vi "DCIR_run_1pulseGene.vi"(6 "3P4S":bool, 7 "Offset%":sgl, 8 "errin":errorcluster, 9 "AmpCharg":dbl, 11 "VisaAlimIn":refnum<visa-resource-name>) -> (0 "errout":errorcluster, 1 "PV":string, 2 "DATAout":cluster{"Rch":dbl, "A ch":dbl, "max":dbl}, 3 "VisaAlimOut":refnum<visa-resource-name>, 4 "Out":T1, 5 "Cell et DCIR ok":bool)   [LabVIEW 2020]
uses:
  <userlib>/PCAN Basic/Controls/BaudrateEenum.ctl
  <userlib>/PCAN Basic/Controls/Channel.ctl
  Param_Stack.vi
  ctrl glo/VG_progressBar.vi
  <instrlib>/IT6000C/IT6000C.lvlib
  <userlib>/Alex_Peak_lib/PEAK_lib_ALEX.lvlib
  <userlib>/PCAN Basic/PCANBasic.lvlib
panel:
  out "isPASS?":bool
  out "Rcharge":dbl
  out "Rmax":dbl
  out "V gamme":bool
  in  "stop":bool
  out "Booléen":bool
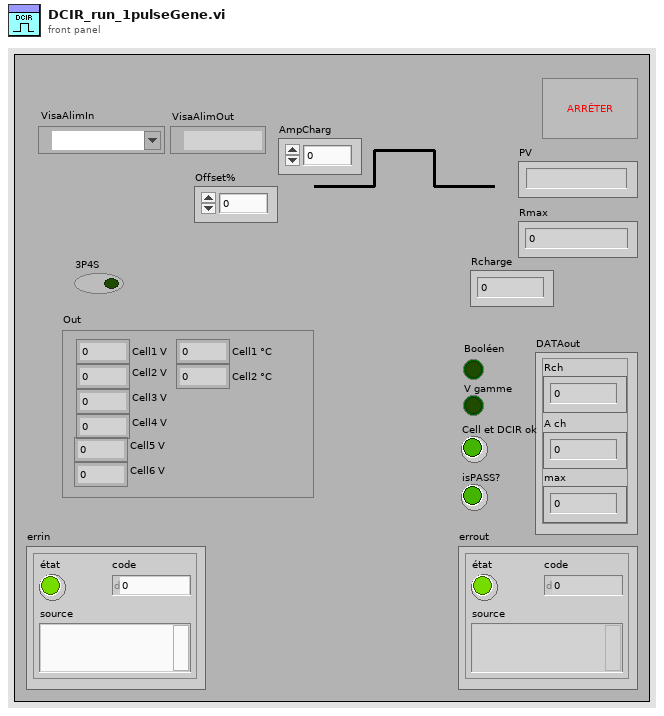
[diagram p1: front panel]
types:
  T1 = cluster{"Cell1 V":sgl, "Cell2 V":sgl, "Cell3 V":sgl, "Cell4 V":sgl, "Cell1 °C":sgl, "Cell2 °C":sgl, "Cell5 V":sgl, "Cell6 V":sgl}
  T2 = typedef "PCANBasic.lvlib/Channel.ctl" = enum16{"PCAN_NONEBUS", "not used1", "not used2", "not used3", "not used4", "not used5", "not used6", "not used7", "not used8", "not used9", "not used10", "not used11", "not used12", "not used13", "not used14", "not used15", "not used16", "not used17", "not used18", "not used19", "not used20", "not used21", "not used22", "not used23", "not used24", "not used25", "not used26", "not used27", "not used28", "not used29", "not used30", "not used31", "not used32", "PCAN_ISABUS1", "PCAN_ISABUS2", "PCAN_ISABUS3", "PCAN_ISABUS4", "PCAN_ISABUS5", "PCAN_ISABUS6", "PCAN_ISABUS7", "PCAN_ISABUS8", "not used41", "not used42", "not used43", "not used44", "not used45", "not used46", "not used47", "not used48", "PCAN_DNGBUS1", "not used50", "not used51", "not used52", "not used53", "not used54", "not used55", "not used56", "not used57", "not used58", "not used59", "not used60", "not used61", "not used62", "not used63", "not used64", "PCAN_PCIBUS1", "PCAN_PCIBUS2", "PCAN_PCIBUS3", "PCAN_PCIBUS4", "PCAN_PCIBUS5", "PCAN_PCIBUS6", "PCAN_PCIBUS7", "PCAN_PCIBUS8", "not used73", "not used74", "not used75", "not used76", "not used77", "not used78", "not used79", "not used80", "PCAN_USBBUS1", "PCAN_USBBUS2", "PCAN_USBBUS3", "PCAN_USBBUS4", "PCAN_USBBUS5", "PCAN_USBBUS6", "PCAN_USBBUS7", "PCAN_USBBUS8", "Not used89", "Not used90", "Not used91", "Not used92", "Not used93", "Not used94", "Not used95", "Not used96", "PCAN_PCCBUS1", "PCAN_PCCBUS2"}
  T3 = typedef "PCANBasic.lvlib/BaudrateEenum.ctl" = enum16{"CAN_Baud_1M", "CAN_Baud_800K", "CAN_BAUD_500K", "CAN_BAUD_250K", "CAN_BAUD_125K", "CAN_BAUD_100K", "CAN_BAUD_95K", "CAN_BAUD_83K", "CAN_BAUD_50K", "CAN_BAUD_47K", "CAN_BAUD_33K", "CAN_BAUD_20K", "CAN_BAUD_10K", "CAN_BAUD_5K", "User Baudrate"}
  T4 = cluster{"Cell1 °C":sgl, "Cell2 °C":sgl, "Cell3 °C":sgl, "Cell4 °C":sgl, "Cell_1_Volt":sgl, "Cell_2_Volt":sgl, "Cell_3_Volt":sgl, "Cell_4_Volt":sgl}
  T5 = cluster{"ID":u32, "MSGTYPE":u8, "LEN":u8, "DATA[0]":u8, "DATA[1]":u8, "DATA[2]":u8, "DATA[3]":u8, "DATA[4]":u8, "DATA[5]":u8, "DATA[6]":u8, "DATA[7]":u8}
  T6 = cluster{"Cell_1_Temperature":sgl, "Cell_1_Voltage":sgl, "Cell_2_Temperature":sgl, "Cell_2_Voltage":sgl}
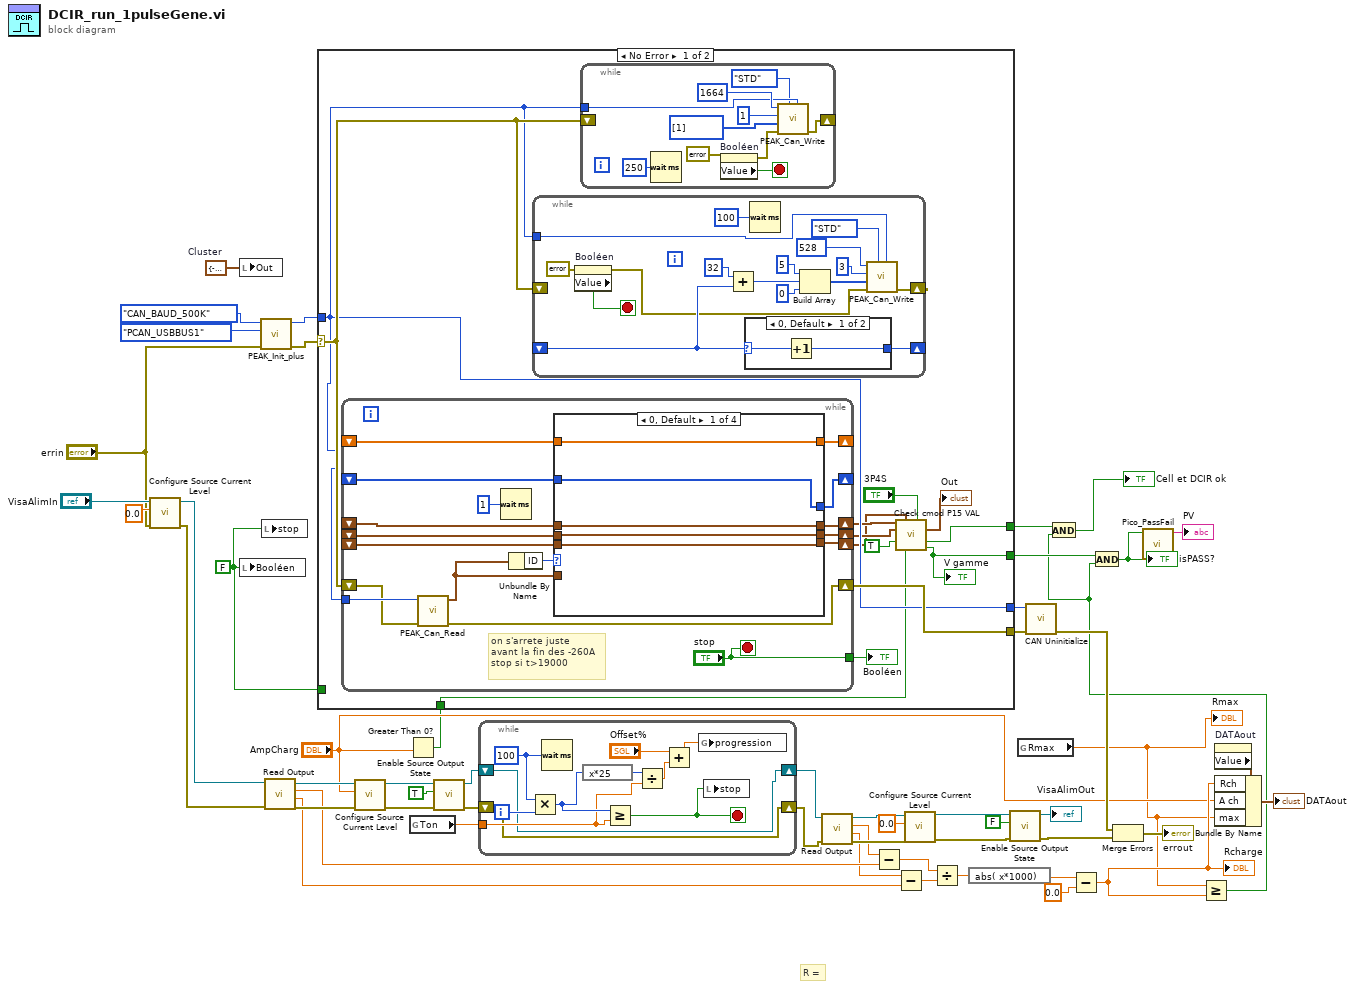
[diagram p0: block diagram]
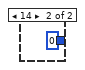
[diagram p2: hidden frame]
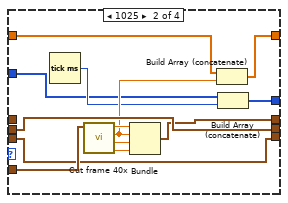
[diagram p3: hidden frame]
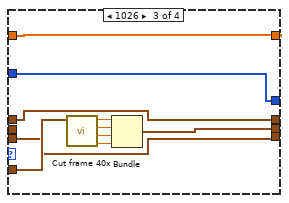
[diagram p4: hidden frame]
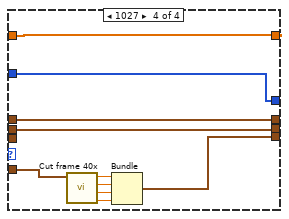
[diagram p5: hidden frame]
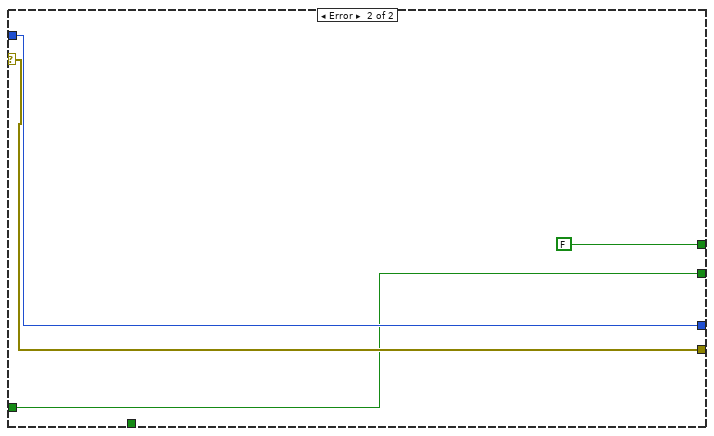
[diagram p6: hidden frame]
diagram:
  w46 = FALSE ("Booléen")
  w7 = T4 {"Cell1 °C"=-1.0, "Cell2 °C"=-1.0, "Cell3 °C"=-1.0, "Cell4 °C"=-1.0, "Cell_1_Volt"=-1.0, "Cell_2_Volt"=-1.0, "Cell_3_Volt"=-1.0, "Cell_4_Volt"=-1.0}  # Cluster
  # "R ="
  n1 = call <instrlib>:"Configure Source Current Level.vi"("error in (no error)"="errin", "Value(0)"=0.0, "VISA resource name"="VisaAlimIn") -> ("error out"=w15:errorcluster, "VISA resource name out"=w16:refnum<visa-resource-name>)  [unwired: 7 in]
  n2 = local write "Out"(w7) -> ()
  n3 = local write "Booléen"(w46) -> ()
  n4 = call <userlib>:"PEAK_Init_plus.vi"("errin"="errin", "Channel"=Channel."PCAN_USBBUS1", "BTR0BTR1"=BaudrateEenum."CAN_BAUD_500K") -> ("errout"=w45:errorcluster, "Channel out"=w44:T2)  [unwired: 7 in]
  n5 = local write "stop"(w46) -> ()
  n6 = call <instrlib>:"Read Output.vi"("error in (no error)"=w15, "VISA resource name"=w16) -> ("error out"=w42:errorcluster, "Actual Current Level (A)"=w25:dbl, "Actual Voltage Level (V)"=w27:dbl, "VISA resource name out"=w41:refnum<visa-resource-name>)  [unwired: 6 in]
  n7 = call <instrlib>:"Configure Source Current Level.vi"("error in (no error)"=w42, "Value(0)"="AmpCharg", "VISA resource name"=w41) -> ("error out"=w39:errorcluster, "VISA resource name out"=w38:refnum<visa-resource-name>)  [unwired: 7 in]
  n8 = Greater Than 0?(x="AmpCharg") -> (x > 0?=w5:bool)
  n9 = case shown="No Error" w45 {
    selector: w45 -> [w67 w155]
    tunnel: w44 -> [w65 w154]
    tunnel: [w66 w155] -> w49
    tunnel: [w65 w154] -> w50
    tunnel: w46 -> [_ w153]
    tunnel: [w60 w153] -> w21
    tunnel: [w59 FALSE ("ok global")] -> w10
    tunnel: w5 -> [w55 _]
    frame No Error {
      n10 = while {
        shift-right: [w106] -> w66
        shift-left: w67 -> [w111]
        shift-right: [w104] -> w63
        shift-left: _ -> [w108]
        shift-right: [w105] -> w62
        shift-left: _ -> [w107]
        tunnel: w65 -> [w112]
        tunnel: ["stop"] -> w64
        shift-right: [w101] -> _
        shift-left: _ -> [w102]
        shift-right: [w99] -> _
        shift-left: _ -> [w100]
        shift-right: [w98] -> w58
        shift-left: _ -> [w97]
        stop <- "stop" stop-if-true
        # "on s'arrete juste \navant la fin des -260A\nstop si t>19000"
        n11 = call <userlib>:"PEAK_Can_Read.vi"("errin"=w111, "Channel out"=w112) -> ("errout"=w106:errorcluster, "MessageBuffer out"=w110:T5)  [unwired: 7 in, 1 out]
        n12 = Wait (ms)(milliseconds to wait=u32 1 ("attente (ms)")) -> ()  [unwired: 1 out]
        n13 = Unbundle By Name(w110) -> ("ID"=w109:u32)
        n14 = case shown="0, Default" w109 {
          tunnel: w110 -> [_ w128 w136 w147]
          tunnel: [w118 w126 w135 w146] -> w104
          tunnel: [w117 w127 w137 w143] -> w105
          tunnel: w108 -> [w118 _ w135 w146]
          tunnel: w107 -> [w117 w127 _ w143]
          tunnel: w102 -> [w116 w125 w134 w145]
          tunnel: [w116 w124 w134 w145] -> w101
          tunnel: w100 -> [w115 w121 w133 w144]
          tunnel: [w115 w120 w133 w144] -> w99
          tunnel: [w114 w119 w132 w142] -> w98
          tunnel: w97 -> [w114 w119 w132 _]
          frame 0, Default {
          }
          frame 1025 {
            n15 = Tick Count (ms)() -> (millisecond timer value=w122:u32)
            n16 = call "Cut frame 40x.vi"("MessageBuffer out"=w128) -> ("Cell_2_Voltage"=w129:sgl, "Cell_2_Temperature"=w130:sgl, "Cell_1_Voltage"=w123:sgl, "Cell_1_Temperature"=w131:sgl)  [unwired: 7 in]
            n17 = Bundle("Cell_1_Temperature"=w131, "Cell_1_Voltage"=w123, "Cell_2_Temperature"=w130, "Cell_2_Voltage"=w129) -> (w126:T6)  [unwired: 1 in]
            n18 = Build Array (concatenate)(w125, w123) -> (w124:sgl[])
            n19 = Build Array (concatenate)(w121, w122) -> (w120:u32[])
          }
          frame 1026 {
            n20 = call "Cut frame 40x.vi"("MessageBuffer out"=w136) -> ("Cell_2_Voltage"=w138:sgl, "Cell_2_Temperature"=w139:sgl, "Cell_1_Voltage"=w140:sgl, "Cell_1_Temperature"=w141:sgl)  [unwired: 7 in]
            n21 = Bundle("Cell_1_Temperature"=w141, "Cell_1_Voltage"=w140, "Cell_2_Temperature"=w139, "Cell_2_Voltage"=w138) -> (w137:T6)  [unwired: 1 in]
          }
          frame 1027 {
            n22 = call "Cut frame 40x.vi"("MessageBuffer out"=w147) -> ("Cell_2_Voltage"=w148:sgl, "Cell_2_Temperature"=w149:sgl, "Cell_1_Voltage"=w150:sgl, "Cell_1_Temperature"=w151:sgl)  [unwired: 7 in]
            n23 = Bundle("Cell_1_Temperature"=w151, "Cell_1_Voltage"=w150, "Cell_2_Temperature"=w149, "Cell_2_Voltage"=w148) -> (w142:T6)  [unwired: 1 in]
          }
        }
      }
      "Booléen" <- w64
      n24 = while {
        tunnel: w65 -> [w78]
        shift-right: [w93] -> _
        shift-left: _ -> [w92]
        shift-right: [w91] -> _
        shift-left: w67 -> [_]
        stop <- w89 stop-if-true
        n25 = property on="Booléen" class="Bool (strict)"(error in=errorcluster {"status"=FALSE, "code"=0, "source"=""} ("entrée d'erreur (pas d'erreur)")) -> (error out=w90:errorcluster, "Value"=w89:bool)  [unwired: 1 in, 1 out]
        n26 = Add(x=u8 32, y=w92) -> (x+y=w84:i32)
        n27 = case shown="0, Default" w92 {
          selector: w92 -> [w95 _]
          tunnel: [w94 0] -> w93
          frame 0, Default {
            n28 = Increment(x=w95) -> (x+1=w94:i32)
          }
          frame 14 {
          }
        }
        n29 = Wait (ms)(milliseconds to wait=u32 100 ("attente (ms)")) -> ()  [unwired: 1 out]
        n30 = Build Array(u8 5 ("élément"), w84, u8 0 ("élément")) -> (w83:i32[])
        n31 = call <userlib>:"PEAK_Can_Write.vi"("CAN Handle"=w78, "MSG type"=enum8{"STD", "RTR", "XTD", "XTD RTR", "STATUS"}."STD", "errin"=w90, "CAN Data"=w83, "DLC (8)"=u8 3, "Identifier"=u32 528) -> ("errout"=w91:errorcluster)  [unwired: 5 in]
      }
      n32 = while {
        tunnel: w65 -> [w70]
        shift-right: [w74] -> _
        shift-left: w67 -> [_]
        stop <- w77 stop-if-true
        n33 = Wait (ms)(milliseconds to wait=u32 250 ("attente (ms)")) -> ()  [unwired: 1 out]
        n34 = property on="Booléen" class="Bool (strict)"(error in=errorcluster {"status"=FALSE, "code"=0, "source"=""} ("entrée d'erreur (pas d'erreur)")) -> (error out=w73:errorcluster, "Value"=w77:bool)  [unwired: 1 in, 1 out]
        n35 = call <userlib>:"PEAK_Can_Write.vi"("CAN Handle"=w70, "MSG type"=enum8{"STD", "RTR", "XTD", "XTD RTR", "STATUS"}."STD", "errin"=w73, "CAN Data"=u8[] [1], "DLC (8)"=u8 1, "Identifier"=u32 1664) -> ("errout"=w74:errorcluster)  [unwired: 5 in]
      }
      n36 = call "Check cmod P15 VAL.vi"("Cell 1 et 2"=w63, "Cell 5 et 6"=w58, "3P4S"="3P4S", "Cell 3 et 4"=w62, "intra?"=TRUE, "isPos?"=w55) -> ("Out"=→"Out":T1, "ok global"=w59:bool, "V gamme"=w60:bool)  [unwired: 5 in, 2 out]
      "V gamme" <- w60
    }
    frame Error {
    }
  }
  n37 = global read "Param_Stack.vi" "Ton"() -> (w1:dbl)
  n38 = call <instrlib>:"Enable Source Output State.vi"("error in (no error)"=w39, "Enable(True)"=TRUE, "VISA resource name"=w38) -> ("error out"=w14:errorcluster, "VISA resource name out"=w12:refnum<visa-resource-name>)  [unwired: 7 in]
  n39 = while {
    tunnel: w1 -> [w161]
    shift-right: [w159] -> w11
    shift-left: w12 -> [w159]
    shift-right: [w160] -> w13
    shift-left: w14 -> [w160]
    i -> [w166]
    stop <- w164 stop-if-true
    w165 = u32 100 ("attente (ms)")
    n40 = Multiply(x=w165, y=w166) -> (x*y=w162:u32)
    n41 = Wait (ms)(milliseconds to wait=w165) -> ()  [unwired: 1 out]
    n42 = expression code="x*25"(w162) -> (w163:u32)
    n43 = Greater Or Equal?(x=w162, y=w161) -> (x >= y?=w164:bool)
    n44 = Divide(x=w163, y=w161) -> (x/y=w158:dbl)
    n45 = Add(x="Offset%", y=w158) -> (x+y=w156:dbl)
    n46 = global write "VG_progressBar.vi" "progression"(w156) -> ()
    n47 = local write "stop"(w164) -> ()
  }
  n48 = call <instrlib>:"Read Output.vi"("error in (no error)"=w13, "VISA resource name"=w11) -> ("error out"=w36:errorcluster, "Actual Current Level (A)"=w26:dbl, "Actual Voltage Level (V)"=w28:dbl, "VISA resource name out"=w35:refnum<visa-resource-name>)  [unwired: 6 in]
  n49 = Subtract(x=w28, y=w27) -> (x-y=w17:dbl)
  n50 = Subtract(x=w26, y=w25) -> (x-y=w31:dbl)
  n51 = call <instrlib>:"Configure Source Current Level.vi"("error in (no error)"=w36, "Value(0)"=0.0, "VISA resource name"=w35) -> ("error out"=w34:errorcluster, "VISA resource name out"=w33:refnum<visa-resource-name>)  [unwired: 7 in]
  n52 = Divide(x=w17, y=w31) -> (x/y=w30:dbl)
  n53 = expression code="abs( x*1000)"(w30) -> (w29:dbl)
  n54 = call <instrlib>:"Enable Source Output State.vi"("error in (no error)"=w34, "Enable(True)"=FALSE, "VISA resource name"=w33) -> ("error out"=w24:errorcluster, "VISA resource name out"=→"VisaAlimOut":refnum<visa-resource-name>)  [unwired: 7 in]
  n55 = global read "Param_Stack.vi" "Rmax"() -> (w4:dbl)
  "Rmax" <- w4
  n56 = call <userlib>:"CAN Uninitialize.vi"("error in (no error)"=w49, "Channel"=w50) -> ("error out"=w47:errorcluster)  [unwired: 7 in, 2 out]
  n57 = Subtract(x=w29, y=0.0) -> (x-y=w18:dbl)
  "Rcharge" <- w18
  n58 = Merge Errors(w47, w24) -> (→"errout":errorcluster)
  n59 = Greater Or Equal?(x=w4, y=w18) -> (x >= y?=w9:bool)
  n60 = And(x=w10, y=w9) -> (x .and. y?=→"Cell et DCIR ok":bool)
  n61 = And(x=w21, y=w9) -> (x .and. y?=w20:bool)
  "isPASS?" <- w20
  n62 = call "Pico_PassFail.vi"("Booléen"=w20) -> ("Vout"=→"PV":string)  [unwired: 10 in]
  n63 = property on="DATAout" class="Clust (strict)"() -> ("Value"=w52:cluster{"Rch":dbl, "A ch":dbl, "max":dbl})  [unwired: 2 in, 2 out]
  n64 = Bundle By Name(cluster=w52, "Rch"=w18, "A ch"="AmpCharg", "max"=w4) -> (→"DATAout":cluster{"Rch":dbl, "A ch":dbl, "max":dbl})
